vi "Example.vi"() -> ()   [LabVIEW 2017]
panel:
  out "Alarm Or Error":bool
  out "读取缓冲区 4":string
  out "读取缓冲区 3":string
  out "Position":i32
  out "读取缓冲区":string
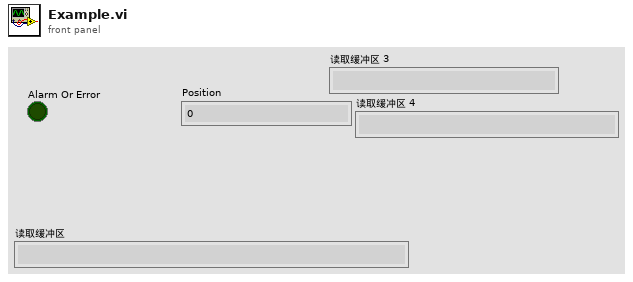
[diagram p1: front panel]
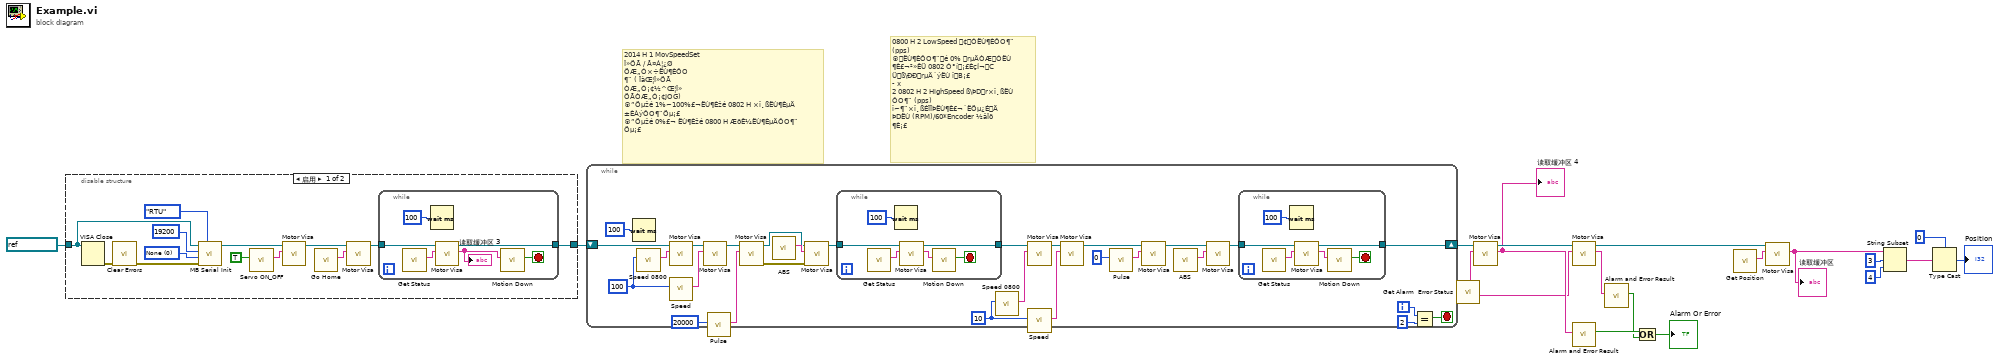
[diagram p0: block diagram]
diagram:
  # "2014 H 1 MovSpeedSet\nÎ»ÖÃ / Å¤Á¦¿Ø\nÖÆ„Ó×÷ËÙ¶ÈÔO\n¶¨ ( ÏàŒ¦Î»ÖÃ\nÒÆ„Ó¡¢½^Œ¦Î»\nÖÃÒÆ„Ó¡¢JOG)\n®”Öµžé 1%~100%£¬ËÙ¶Èžé 0802 H ×î¸ßËÙ¶ÈµÄ\n±ÈÀýÔO¶¨Öµ¡£\n®”Öµžé 0%£¬ ËÙ¶Èžé 0800 H ÆðÊ¼ËÙ¶ÈµÄÔO¶¨\nÖµ¡£"
  # "0800 H 2 LowSpeed ¢ÓËÙ¶ÈÔO¶¨\n(pps)\n®ËÙ¶ÈÔO¶¨é 0% rµÄÒÆÓËÙ\n¶È£¬²»ÊÜ 0802 Ó°í¡£ÈçÍ¬C\nÜß\\ÐÐrµÄ´ýËÙ îB¡£\n- x\n2 0802 H 2 HighSpeed ß\\ÞDr×î¸ßËÙ\nÔO¶¨ (pps)\nî~¶¨×î¸ßÉÏÏÞËÙ¶È£¬´ËÖµ¿ÉÄ\nÞDËÙ (RPM)/60*Encoder ½âÎö\n¶È¡£"
  n1 = disable-structure shown="启用" {
    disable-tunnel: refnum<visa-resource-name> "COM10" ("VISA resource name") -> [w29 w39]
    disable-tunnel: [w21 w39] -> w17
    frame Enabled {
      w30 = u16 0 items=["None", "Odd", "Even", "Mark", "Space"] ("Parity")
      n2 = VISA Close(VISA resource name=w29) -> (error out=w28:errorcluster)  [unwired: 1 in]
      n3 = call <vilib>:"Clear Errors.vi"("error in (no error)"=w28) -> ("error out"=w27:errorcluster)  [unwired: 5 in, 1 out]
      n4 = call "MB Serial Init.vi"("Mode"=enum16{"RTU", "ASCII"}."RTU", "error in (no error)"=w27, "Parity"=w30, "Baud Rate"=u32 19200, "VISA resource name"=w29) -> ("VISA resource name out"=w26:refnum<visa-resource-name>)  [unwired: 5 in, 1 out]
      n5 = call "Servo ON_OFF.vi"("Servo ON/OFF"=TRUE) -> ("Command"=w25:string)  [unwired: 10 in]
      n6 = call "Motor Visa.vi"("Command"=w25, "VISA资源名称"=w26) -> ("VISA资源名称输出"=w20:refnum<visa-resource-name>)  [unwired: 7 in, 2 out]
      n7 = call "Go Home.vi"() -> ("Go Home"=w23:string)  [unwired: 11 in]
      n8 = call "Motor Visa.vi"("Command"=w23, "VISA资源名称"=w20) -> ("VISA资源名称输出"=w22:refnum<visa-resource-name>)  [unwired: 7 in, 2 out]
      n9 = while {
        tunnel: w22 -> [w37]
        tunnel: [w33] -> w21
        stop <- w35 stop-if-true
        n10 = call "Get Status.vi"() -> ("Command"=w38:string)  [unwired: 11 in]
        n11 = Wait (ms)(milliseconds to wait=u32 100 ("等待时间（毫秒）")) -> ()  [unwired: 1 out]
        n12 = call "Motor Visa.vi"("Command"=w38, "VISA资源名称"=w37) -> ("读取缓冲区"=w36:string, "VISA资源名称输出"=w33:refnum<visa-resource-name>)  [unwired: 7 in, 1 out]
        "读取缓冲区 3" <- w36
        n13 = call "Motion Down.vi"("Command"=w36) -> ("Motion Down"=w35:bool)  [unwired: 10 in]
      }
    }
    frame Disabled {
    }
  }
  n14 = while {
    shift-right: [w52] -> w10
    shift-left: w17 -> [w63]
    i -> [w51]
    stop <- w50 stop-if-true
    w41 = 10 ("Speed1")
    w43 = 100 ("Speed1")
    n15 = Wait (ms)(milliseconds to wait=u32 100 ("等待时间（毫秒）")) -> ()  [unwired: 1 out]
    n16 = call "Speed 0800.vi"("Speed"=w43) -> ("Command"=w42:string)  [unwired: 10 in]
    n17 = call "Motor Visa.vi"("Command"=w42, "VISA资源名称"=w63) -> ("VISA资源名称输出"=w60:refnum<visa-resource-name>)  [unwired: 7 in, 2 out]
    n18 = call "Speed.vi"("Speed"=w43) -> ("速度"=w58:string)  [unwired: 10 in]
    n19 = call "Motor Visa.vi"("Command"=w58, "VISA资源名称"=w60) -> ("VISA资源名称输出"=w59:refnum<visa-resource-name>)  [unwired: 7 in, 2 out]
    n20 = call "Pulse.vi"("Pulse"=20000) -> ("Pulse"=w67:string)  [unwired: 10 in]
    n21 = call "Motor Visa.vi"("Command"=w67, "VISA资源名称"=w59) -> ("错误输出"=w64:errorcluster, "VISA资源名称输出"=w65:refnum<visa-resource-name>)  [unwired: 7 in, 1 out]
    n22 = call "ABS.vi"() -> ("绝对模式"=w66:string)  [unwired: 11 in]
    n23 = call "Motor Visa.vi"("错误输入（无错误）"=w64, "Command"=w66, "VISA资源名称"=w65) -> ("VISA资源名称输出"=w62:refnum<visa-resource-name>)  [unwired: 6 in, 2 out]
    n24 = while {
      tunnel: w62 -> [w78]
      tunnel: [w74] -> w45
      stop <- w76 stop-if-true
      n25 = call "Get Status.vi"() -> ("Command"=w79:string)  [unwired: 11 in]
      n26 = Wait (ms)(milliseconds to wait=u32 100 ("等待时间（毫秒）")) -> ()  [unwired: 1 out]
      n27 = call "Motor Visa.vi"("Command"=w79, "VISA资源名称"=w78) -> ("读取缓冲区"=w77:string, "VISA资源名称输出"=w74:refnum<visa-resource-name>)  [unwired: 7 in, 1 out]
      n28 = call "Motion Down.vi"("Command"=w77) -> ("Motion Down"=w76:bool)  [unwired: 10 in]
    }
    n29 = call "Speed 0800.vi"("Speed"=w41) -> ("Command"=w40:string)  [unwired: 10 in]
    n30 = call "Motor Visa.vi"("Command"=w40, "VISA资源名称"=w45) -> ("VISA资源名称输出"=w46:refnum<visa-resource-name>)  [unwired: 7 in, 2 out]
    n31 = call "Speed.vi"("Speed"=w41) -> ("速度"=w47:string)  [unwired: 10 in]
    n32 = call "Motor Visa.vi"("Command"=w47, "VISA资源名称"=w46) -> ("VISA资源名称输出"=w44:refnum<visa-resource-name>)  [unwired: 7 in, 2 out]
    n33 = call "Pulse.vi"("Pulse"=0) -> ("Pulse"=w54:string)  [unwired: 10 in]
    n34 = call "Motor Visa.vi"("Command"=w54, "VISA资源名称"=w44) -> ("VISA资源名称输出"=w55:refnum<visa-resource-name>)  [unwired: 7 in, 2 out]
    n35 = call "ABS.vi"() -> ("绝对模式"=w57:string)  [unwired: 11 in]
    n36 = call "Motor Visa.vi"("Command"=w57, "VISA资源名称"=w55) -> ("VISA资源名称输出"=w53:refnum<visa-resource-name>)  [unwired: 7 in, 2 out]
    n37 = while {
      tunnel: w53 -> [w72]
      tunnel: [w68] -> w52
      stop <- w70 stop-if-true
      n38 = call "Get Status.vi"() -> ("Command"=w73:string)  [unwired: 11 in]
      n39 = Wait (ms)(milliseconds to wait=u32 100 ("等待时间（毫秒）")) -> ()  [unwired: 1 out]
      n40 = call "Motor Visa.vi"("Command"=w73, "VISA资源名称"=w72) -> ("读取缓冲区"=w71:string, "VISA资源名称输出"=w68:refnum<visa-resource-name>)  [unwired: 7 in, 1 out]
      n41 = call "Motion Down.vi"("Command"=w71) -> ("Motion Down"=w70:bool)  [unwired: 10 in]
    }
    n42 = Equal?(x=w51, y=2) -> (x = y?=w50:bool)
  }
  n43 = call "Get Alarm  Error Status.vi"() -> ("AlarmStatus"=w1:string, "ErrorStatus"=w2:string)  [unwired: 10 in]
  n44 = call "Motor Visa.vi"("Command"=w2, "VISA资源名称"=w10) -> ("读取缓冲区"=w6:string, "VISA资源名称输出"=w9:refnum<visa-resource-name>)  [unwired: 7 in, 1 out]
  "读取缓冲区 4" <- w6
  n45 = call "Motor Visa.vi"("Command"=w1, "VISA资源名称"=w9) -> ("读取缓冲区"=w4:string, "VISA资源名称输出"=w8:refnum<visa-resource-name>)  [unwired: 7 in, 1 out]
  n46 = call "Alarm and Error Result.vi"("Command"=w6) -> ("Alarm or Error"=w5:bool)  [unwired: 10 in]
  n47 = call "Alarm and Error Result.vi"("Command"=w4) -> ("Alarm or Error"=w3:bool)  [unwired: 10 in]
  n48 = Or(x=w5, y=w3) -> (x .or. y?=→"Alarm Or Error":bool)
  n49 = call "Get Position.vi"() -> ("Position"=w18:string)  [unwired: 11 in]
  n50 = call "Motor Visa.vi"("Command"=w18, "VISA资源名称"=w8) -> ("读取缓冲区"=w16:string)  [unwired: 7 in, 2 out]
  "读取缓冲区" <- w16
  n51 = String Subset(string=w16, offset (0)=3 ("偏移量(0)"), length (rest)=4 ("长度（剩余）")) -> (substring=w13:string)
  n52 = Type Cast(type=0, x=w13) -> (*(type *) &x=→"Position":i32)
